vi "子VI.vi"(1 "b":dbl, 2 "c":dbl, 3 "a":dbl) -> (0 "数值":dbl)   [LabVIEW 2018]
doc: "这个程序是进行y=a^3+b^2+c"
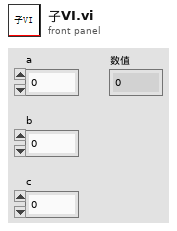
[diagram p1: front panel]
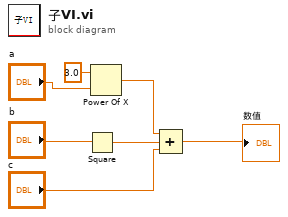
[diagram p0: block diagram]
diagram:
  n1 = Square(x="b") -> (x^2=w5:dbl)
  n2 = Power Of X(1:"a", 2:3.0 ("y")) -> (0:w6:dbl)
  n3 = Compound Arithmetic op=ADD(w6, w5, "c") -> (→"数值":dbl)
